vi "IR STIM Manual (SubVI).vi"(9 "IR Stimulus Settings":cluster{"X":dbl, "Y":dbl, "TON (ms)":dbl}[](array[cluster])=[{"X"=600.0, "Y"=600.0, "TON (ms)"=12.5}, {"X"=1200.0, "Y"=1200.0, "TON (ms)"=12.5}, {"X"=1800.0, "Y"=1800.0, "TON (ms)"=12.5}, {"X"=2400.0, "Y"=2400.0, "TON (ms)"=12.5}] {"TON (ms)" step=0.1 format="%#.1f"; "Y" step=1.0 format="%#.0f"; "X" step=1.0 format="%#.0f"}, 10 "Cycle Time (ms)":i32=50) -> (3 "DAQ Data":dbl[][](array[numeric]))   [LabVIEW 2015]
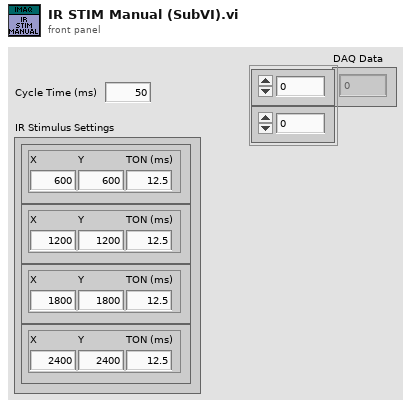
[diagram p1: front panel]
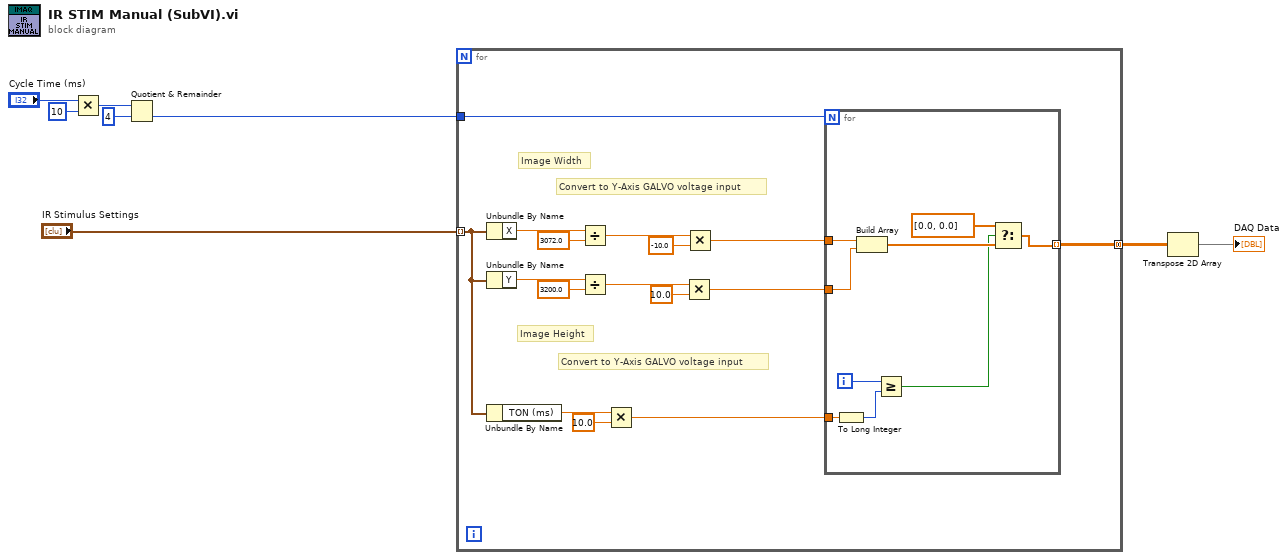
[diagram p0: block diagram]
diagram:
  n1 = Multiply(x="Cycle Time (ms)", y=10) -> (x*y=w4:i32)
  n2 = Quotient & Remainder(x=w4, y=4) -> (floor(x/y)=w7:i32)  [unwired: 1 out]
  n3 = for {
    tunnel: "IR Stimulus Settings" -> [w24] mode=indexing
    tunnel: [w10] -> w2 mode=concatenating
    tunnel: w7 -> [w9]
    # "Convert to Y-Axis GALVO voltage input"
    # "Convert to Y-Axis GALVO voltage input"
    # "Image Height"
    # "Image Width"
    n4 = Unbundle By Name(w24) -> ("X"=w23:dbl)
    n5 = Unbundle By Name(w24) -> ("Y"=w20:dbl)
    n6 = Unbundle By Name(w24) -> ("TON (ms)"=w14:dbl)
    n7 = Divide(x=w23, y=3072.0) -> (x/y=w19:dbl)
    n8 = Divide(x=w20, y=3200.0) -> (x/y=w16:dbl)
    n9 = Multiply(x=w14, y=10.0) -> (x*y=w11:dbl)
    n10 = Multiply(x=w16, y=10.0) -> (x*y=w12:dbl)
    n11 = Multiply(x=w19, y=-10.0) -> (x*y=w13:dbl)
    n12 = for {
      N: w9 -> [_]
      tunnel: w13 -> [w33]
      tunnel: w12 -> [w32]
      tunnel: [w30] -> w10 mode=indexing
      tunnel: w11 -> [w28]
      i -> [w29]
      n13 = To Long Integer(number=w28) -> (32bit integer=w27:i32)
      n14 = Build Array(w33, w32) -> (w31:dbl[])
      n15 = Greater Or Equal?(x=w29, y=w27) -> (x >= y?=w26:bool)
      n16 = Select(t=dbl[] [0.0, 0.0], s=w26, f=w31) -> (s? t:f=w30:dbl[])
    }
  }
  n17 = Transpose 2D Array(2D array=w2) -> (transposed array=→"DAQ Data":dbl[][])
